vi "Parse Light IDs.vi"(8 "Error In":errorcluster, 10 "Light JSON":string="{\"1\":{\"name\": \"Hue Lamp\"},\"2\":{\"name\": \"Hue Lamp 1\"},\"3\":{\"name\": \"Hue Lamp 2\"}}") -> (0 "Error Out":errorcluster, 2 "Light IDs":i32[](array[numeric]))   [LabVIEW 2013, in "LVH-Hue.lvlib"]
uses:
  LVH-Hue.lvlib
  <vilib>/regexp/Match Regular Expression.xnode
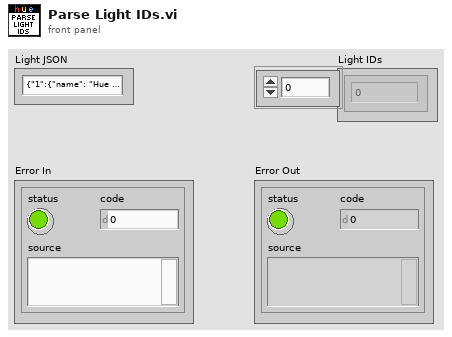
[diagram p1: front panel]
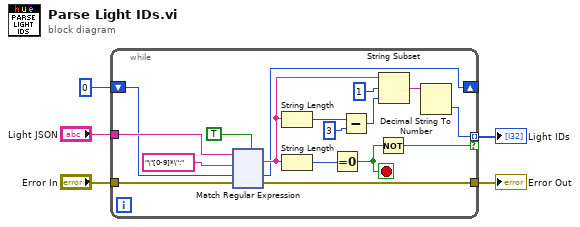
[diagram p0: block diagram]
diagram:
  n1 = while {
    tunnel: "Light JSON" -> [w21]
    shift-right: [w9] -> _
    shift-left: 0 ("y") -> [w14]
    tunnel: "Error In" -> [w13]
    tunnel: [w12] -> w1
    tunnel: [w6] -> w3 mode=indexing if=w7
    stop <- w8 stop-if-true
    n2 = xnode "Match Regular Expression"("input string"=w21, "regular expression"="\"[0-9]*\":", "offset (0)"=w14, "error in"=w13, "multiline? (F)"=TRUE) -> ("whole match"=w11:string, "offset past match"=w9:i32, "error out"=w12:errorcluster)  [unwired: 1 in, 2 out]
    n3 = String Length(string=w11) -> (length=w18:i32)
    n4 = String Length(string=w11) -> (length=w10:i32)
    n5 = Equal To 0?(x=w10) -> (x = 0?=w8:bool)
    n6 = Subtract(x=w18, y=3) -> (x-y=w16:i32)
    n7 = Not(x=w8) -> (.not. x?=w7:bool)
    n8 = String Subset(string=w11, offset (0)=1, length (rest)=w16) -> (substring=w15:string)
    n9 = Decimal String To Number(string=w15) -> (number=w6:i32)  [unwired: 2 in, 1 out]
  }
  "Light IDs" <- w3
  "Error Out" <- w1
